vi "Get Byte Order.vi"(8 "error in (no error)":errorcluster, 11 "CAN Signal in":refnum<class "CAN Signal.lvclass">) -> (0 "error out":errorcluster, 2 "Byte Order":enum16{"Little Endian", "Big Endian"}(ring), 3 "CAN Signal out":refnum<class "CAN Signal.lvclass">)   [LabVIEW 2023, in "CAN Signal.lvclass"]
uses:
  CAN Signal.lvclass
  CAN Signal.lvclass/CAN Signal.ctl
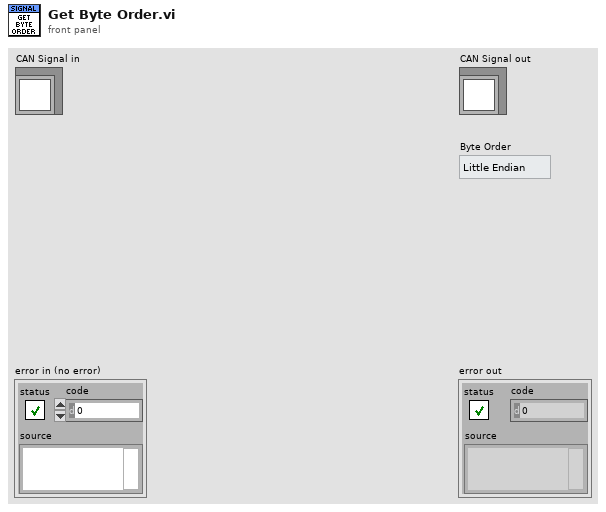
[diagram p1: front panel]
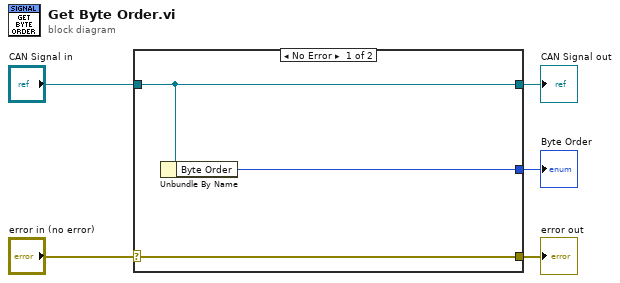
[diagram p0: block diagram]
diagram:
  n1 = case shown="No Error" "error in (no error)" {
    selector: "error in (no error)" -> [w8 w9]
    tunnel: [w8 w9] -> w4
    tunnel: [w7 w10] -> w2
    tunnel: "CAN Signal in" -> [w7 w10]
    tunnel: [w6 _] -> w1
    frame No Error {
      n2 = Unbundle By Name(w7) -> ("Byte Order"=w6:enum16{"Little Endian", "Big Endian"})
    }
    frame Error {
    }
  }
  "error out" <- w4
  "CAN Signal out" <- w2
  "Byte Order" <- w1
